vi "rgb12+.vi"() -> ()   [LabVIEW 2016]
uses:
  <vilib>/LabVIEW Interface for Arduino/LabVIEW Interface for Arduino.lvlib
panel:
  in  "Slide 3":dbl(slide) min=0.0 max=255.0 scale=0.0..255.0
  in  "Slide 2":dbl(slide) min=0.0 max=255.0 scale=0.0..255.0
  in  "Slide":dbl(slide) min=0.0 max=255.0 scale=0.0..255.0
  in  "stop":bool
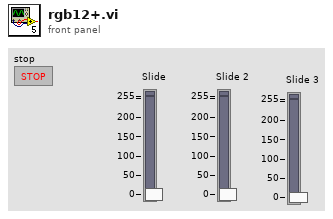
[diagram p1: front panel]
types:
  T1 = typedef "LabVIEW Interface for Arduino.lvlib/Arduino Resource.ctl" = cluster{"VISA resource":refnum<visa-resource-name>, "Board Type":T2, "Connection Type":enum8{"USB / Serial"}, "Bytes Per Packet (15)":u8}
  T2 = typedef "LabVIEW Interface for Arduino.lvlib/Board Type.ctl" = enum16{"Uno", "Dimuelanove w/Atmega 328", "Mega 2560"}
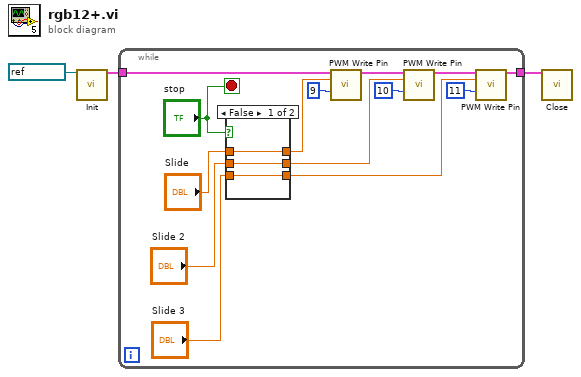
[diagram p0: block diagram]
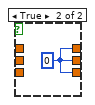
[diagram p2: hidden frame]
diagram:
  n1 = call <vilib>:"Init.vi"("VISA resource"=refnum<visa-resource-name> "COM3") -> ("Arduino Resource"=w3:T1)  [unwired: 17 in, 1 out]
  n2 = while {
    tunnel: w3 -> [w17]
    tunnel: [w14] -> w2
    stop <- "stop" stop-if-true
    n3 = case shown="False" "stop" {
      tunnel: "Slide" -> [w20 _]
      tunnel: "Slide 2" -> [w19 _]
      tunnel: [w20 w21] -> w9
      tunnel: [w19 w21] -> w8
      tunnel: "Slide 3" -> [w18 _]
      tunnel: [w18 w21] -> w5
      frame False {
      }
      frame True {
        w21 = 0
      }
    }
    n4 = call <vilib>:"PWM Write Pin.vi"("Arduino Resource"=w17, "Duty Cycle (0 - 255)"=w9, "PWM Pin (3)"=u8 9) -> ("Arduino Resource"=w16:T1)  [unwired: 11 in, 1 out]
    n5 = call <vilib>:"PWM Write Pin.vi"("Arduino Resource"=w16, "Duty Cycle (0 - 255)"=w8, "PWM Pin (3)"=u8 10) -> ("Arduino Resource"=w15:T1)  [unwired: 11 in, 1 out]
    n6 = call <vilib>:"PWM Write Pin.vi"("Arduino Resource"=w15, "Duty Cycle (0 - 255)"=w5, "PWM Pin (3)"=u8 11) -> ("Arduino Resource"=w14:T1)  [unwired: 11 in, 1 out]
  }
  n7 = call <vilib>:"Close.vi"("Arduino Resource"=w2) -> ()  [unwired: 14 in, 1 out]
